vi "RunningEdgeCount.vi"(1 "Reset Count? (F)":bool, 2 "Input":bool, 4 "Rising Edge? (T)":bool=TRUE) -> (5 "Count":u32)   [LabVIEW 2014]
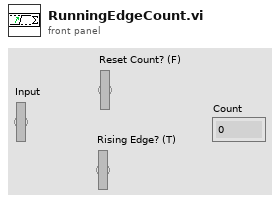
[diagram p1: front panel]
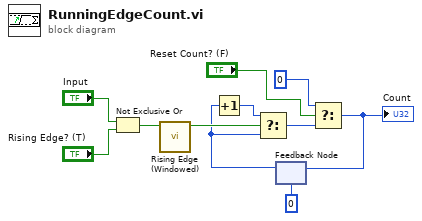
[diagram p0: block diagram]
diagram:
  n1 = Not Exclusive Or(1:"Rising Edge? (T)", 2:"Input") -> (0:w8:bool)
  n2 = call "Rising Edge (Windowed).vi"("Input"=w8) -> ("Rising Edge?"=w7:bool)  [unwired: 10 in]
  n3 = feedback #1(u32 0) -> (w6:u32)
  n4 = Increment(x=w6) -> (x+1=w5:u32)
  n5 = Select(t=w5, s=w7, f=w6) -> (s? t:f=w4:u32)
  n6 = Select(t=u32 0, s="Reset Count? (F)", f=w4) -> (s? t:f=w1:u32)
  "Count" <- w1
  n7 = feedback-in #1(w1) -> ()
